vi "Measure RMS.vi"(2 "Cluster":T1) -> (0 "Waveform Graph":dynamicdata(graph), 1 "RMS":dbl)   [LabVIEW 2015]
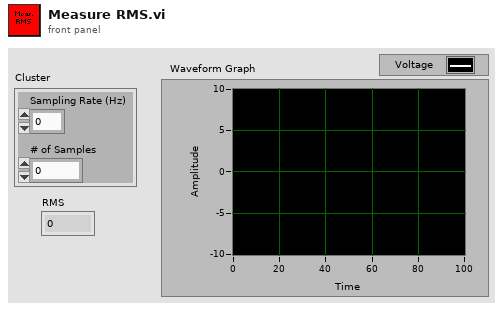
[diagram p1: front panel]
types:
  T1 = cluster{"Sampling Rate (Hz)":dbl, "# of Samples":i32}
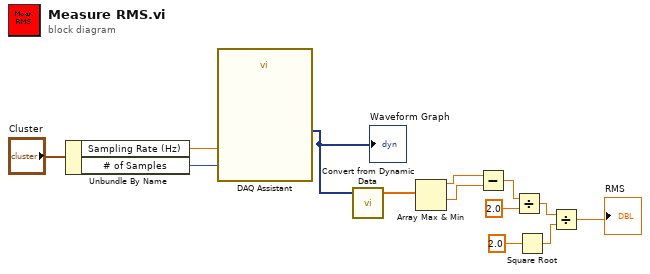
[diagram p0: block diagram]
diagram:
  n1 = Unbundle By Name("Cluster") -> ("Sampling Rate (Hz)"=w2:dbl, "# of Samples"=w1:i32)
  n2 = call "DAQ Assistant"("rate"=w2, "number of samples"=w1) -> ("data"=w13:dynamicdata)  [unwired: 15 in, 2 out]
  "Waveform Graph" <- w13
  n3 = call "Convert from Dynamic Data"("Dynamic Data Type"=w13) -> ("Array"=w12:dbl[])  [unwired: 3 in]
  n4 = Array Max & Min(array=w12) -> (max value=w11:dbl, min value=w10:dbl)  [unwired: 2 out]
  n5 = Subtract(x=w11, y=w10) -> (x-y=w9:dbl)
  n6 = Divide(x=w9, y=2.0) -> (x/y=w7:dbl)
  n7 = Square Root(x=2.0) -> (sqrt(x)=w5:dbl)
  n8 = Divide(x=w7, y=w5) -> (x/y=→"RMS":dbl)
